vi "CameraStateController.vi"(1 "Master State":string) -> ()   [LabVIEW 2019]
doc: "This VI manages the LimeLight pipelines and LimeLight targeting LED mode."
uses:
  dsdata.vi
  sensors.vi
  outputs.vi
  dsinstructions.vi
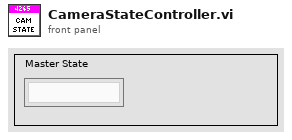
[diagram p1: front panel]
types:
  T1 = enum16{"Boot Up", "Camera Override", "Power Port", "Ball Tracking"}
  T2 = enum16{"Driver Control", "Auto Targeting", "Feeder Station"}
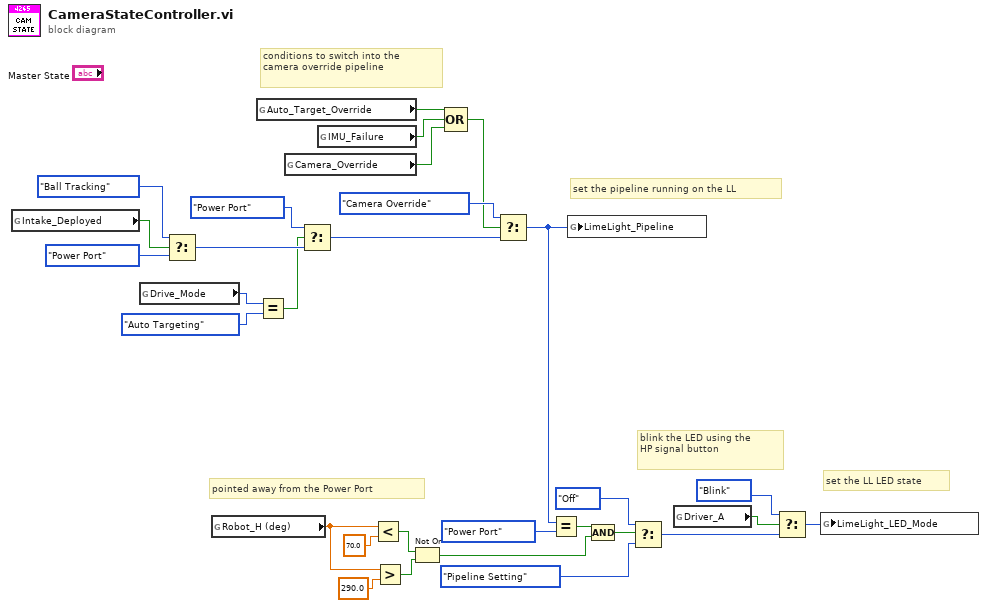
[diagram p0: block diagram]
diagram:
  # "set the LL LED state"
  # "pointed away from the Power Port"
  # "conditions to switch into the \ncamera override pipeline"
  # "set the pipeline running on the LL"
  # "blink the LED using the\nHP signal button"
  n1 = global read "outputs.vi" "Intake_Deployed"() -> (w26:bool)
  n2 = global read "outputs.vi" "Drive_Mode"() -> (w6:T2)
  n3 = Select(t=T1."Ball Tracking", s=w26, f=T1."Power Port") -> (s? t:f=w3:T1)
  n4 = global read "sensors.vi" "Robot_H (deg)"() -> (w12:dbl)
  n5 = global read "dsdata.vi" "Auto_Target_Override"() -> (w30:bool)
  n6 = Equal?(x=w6, y=T2."Auto Targeting") -> (x = y?=w2:bool)
  n7 = global read "dsdata.vi" "Camera_Override"() -> (w28:bool)
  n8 = Select(t=T1."Power Port", s=w2, f=w3) -> (s? t:f=w1:T1)
  n9 = global read "sensors.vi" "IMU_Failure"() -> (w29:bool)
  n10 = Less?(x=w12, y=70.0) -> (x < y?=w13:bool)
  n11 = Greater?(x=w12, y=290.0) -> (0:w14:bool)
  n12 = Not Or(1:w14, 2:w13) -> (0:w8:bool)
  n13 = Compound Arithmetic op=OR(w30, w29, w28) -> (w24:bool)
  n14 = Select(t=T1."Camera Override", s=w24, f=w1) -> (s? t:f=w10:T1)
  n15 = Equal?(x=w10, y=T1."Power Port") -> (x = y?=w11:bool)
  n16 = global write "outputs.vi" "LimeLight_Pipeline"(w10) -> ()
  n17 = Compound Arithmetic op=AND(w11, w8) -> (w23:bool)
  n18 = Select(t=enum16{"Pipeline Setting", "Off", "Blink", "On"}."Off", s=w23, f=enum16{"Pipeline Setting", "Off", "Blink", "On"}."Pipeline Setting") -> (s? t:f=w18:enum16{"Pipeline Setting", "Off", "Blink", "On"})
  n19 = global read "dsinstructions.vi" "Driver_A"() -> (w21:bool)
  n20 = Select(t=enum16{"Pipeline Setting", "Off", "Blink", "On"}."Blink", s=w21, f=w18) -> (s? t:f=w17:enum16{"Pipeline Setting", "Off", "Blink", "On"})
  n21 = global write "outputs.vi" "LimeLight_LED_Mode"(w17) -> ()
